vi "Main.vi"() -> ()   [LabVIEW 2017]
doc: "The myRIO Project template acquires acceleration data from the onboard accelerometer and displays the changes of acceleration values in a waveform chart."
uses:
  <vilib>/myRIO/Instrument Drivers/Onboard IO/AI/typedefs/AI Reference.ctl
  <vilib>/myRIO/Common/Instrument Driver Framework/Utilities/typedefs/myRIO Generic Hardware Reference.ctl
  <vilib>/myRIO/Common/Instrument Driver Framework/Utilities/typedefs/Hardware Version Enum.ctl
  <vilib>/myRIO/Common/Instrument Driver Framework/Utilities/typedefs/myRIO v1.0 Reference.ctl
  <vilib>/myRIO/Common/Instrument Driver Framework/Utilities/typedefs/Generic FPGA Reference.ctl
  <vilib>/myRIO/Common/Instrument Driver Framework/myRIO v1.0/AI/typedefs/AI Channels List.ctl
  <vilib>/myRIO/Common/Instrument Driver Framework/myRIO v1.0/AI/typedefs/AI Channels Enum.ctl
  <vilib>/myRIO/Common/Instrument Driver Framework/Utilities/typedefs/Analog Scaling Constants List.ctl
  <vilib>/myRIO/Common/Instrument Driver Framework/Utilities/typedefs/Analog Scaling Constants.ctl
  <vilib>/userdefined/High Color/nirio_resource_hc.ctl
  <vilib>/myRIO/Instrument Drivers/Onboard IO/DIO/typedefs/DIO Reference.ctl
  <vilib>/myRIO/Common/Instrument Driver Framework/myRIO v1.0/DIO/typedefs/DIO Channels List.ctl
  <vilib>/myRIO/Common/Instrument Driver Framework/myRIO v1.0/DIO/typedefs/DIO Channels Enum.ctl
  <vilib>/myRIO/Common/Instrument Driver Framework/Utilities/vis/Is FPGA Ref Available.vi
  <vilib>/myRIO/Common/Instrument Driver Framework/myRIO v1.0/AI/vis/myRIO v1.1 Open AI.vi
  <vilib>/myRIO/Instrument Drivers/Onboard IO/AI/vis/Read.vi
  <vilib>/Analysis/baseanly.llb/Mean (DBL).vi
  <vilib>/myRIO/Common/Instrument Driver Framework/myRIO v1.0/DIO/vis/myRIO v1.1 Open DIO.vi
  <vilib>/myRIO/Instrument Drivers/Onboard IO/DIO/vis/Write.vi
  <vilib>/myRIO/Common/Instrument Driver Framework/Utilities/vis/Validate Channels.vi
  <vilib>/myRIO/Common/Instrument Driver Framework/myRIO v1.0/AI/vis/myRIO v1.0 Reserve AI.vi
  <vilib>/myRIO/Common/Instrument Driver Framework/myRIO v1.0/DIO/vis/myRIO v1.0 Reserve DIO.vi
  <vilib>/myRIO/Common/Instrument Driver Framework/myRIO v1.0/UART/vis/myRIO v1.0 Close UART.vi
  <vilib>/myRIO/Common/Instrument Driver Framework/myRIO v1.0/AI/vis/myRIO v1.0 Build MUX Configuration AI.vi
  <vilib>/myRIO/Common/Instrument Driver Framework/myRIO v1.0/Resource Manager/vis/myRIO v1.0 Reserve Channel List.vi
  <vilib>/myRIO/Common/Instrument Driver Framework/myRIO v1.0/DIO/vis/myRIO v1.0 Build MUX Configuration DIO.vi
  <vilib>/myRIO/Common/Instrument Driver Framework/myRIO v1.0/Resource Manager/vis/myRIO v1.0 Reserve Channel.vi
  <vilib>/myRIO/Common/Instrument Driver Framework/myRIO v1.0/Resource Manager/vis/myRIO v1.0 Unreserve Channel.vi
  <vilib>/myRIO/Common/Instrument Driver Framework/myRIO v1.0/Resource Manager/vis/myRIO v1.0 Create Configuration List.vi
  <vilib>/myRIO/Common/Instrument Driver Framework/myRIO v1.0/Resource Manager/vis/myRIO v1.0 Build Mutex Name.vi
  <vilib>/Utility/VariantDataType/GetNumericInfo.vi
  <vilib>/Utility/error.llb/Error Cluster From Error Code.vi
  <vilib>/myRIO/Common/Instrument Driver Framework/myRIO v1.0/myRIO v1.1 Open.vi
  <vilib>/myRIO/Common/Instrument Driver Framework/myRIO v1.0/AI/vis/myRIO v1.0 Get Scaling Constants AI.vi
  <vilib>/myRIO/Common/Instrument Driver Framework/Utilities/vis/IO Manager.vi
  <vilib>/myRIO/Common/Instrument Driver Framework/Utilities/vis/Configuration Manager.vi
  <vilib>/myRIO/Common/Instrument Driver Framework/myRIO v1.0/myRIO v1.0 Close.vi
  <vilib>/myRIO/Common/Instrument Driver Framework/myRIO v1.0/AI/vis/myRIO v1.0 Read AI.vi
  <vilib>/myRIO/Common/Instrument Driver Framework/myRIO v1.0/Resource Manager/vis/myRIO v1.0 Configure IO.vi
  <vilib>/myRIO/Common/Instrument Driver Framework/myRIO v1.0/DIO/vis/myRIO v1.0 Write DIO.vi
  <vilib>/myRIO/Common/Instrument Driver Framework/Utilities/vis/FPGA Ref Manager.vi
  <vilib>/myRIO/Common/Instrument Driver Framework/myRIO v1.0/myRIO v1.0 Reset FPGA.vi
  <vilib>/myRIO/Common/Instrument Driver Framework/myRIO v1.0/IRQ/vis/myRIO v1.0 IRQ Info FGV.vi
  <vilib>/myRIO/Common/Instrument Driver Framework/myRIO v1.0/IRQ/vis/myRIO v1.0 Timer IRQ Info FGV.vi
  <vilib>/myRIO/Common/Instrument Driver Framework/myRIO v1.0/IRQ/vis/myRIO v1.0 ISR Agent.vi
  <vilib>/myRIO/Express VI/Onboard IO/AI/AI Express VI.xnode
  <vilib>/myRIO/Instrument Drivers/Onboard IO/AI/vis/myRIO AI Open.xnode
  <vilib>/myRIO/Express VI/Onboard Devices/LED/LED Express VI.xnode
  <vilib>/myRIO/Instrument Drivers/Onboard IO/DIO/vis/myRIO DIO Open.xnode
  <vilib>/myRIO/Instrument Drivers/Utilities/Utilities.lvlib
  <vilib>/myRIO/Instrument Drivers/Onboard IO/AI/AI.lvlib
  <vilib>/Analysis/NI_AALBase.lvlib
  <vilib>/myRIO/Instrument Drivers/Onboard IO/DIO/DIO.lvlib
panel:
  in  "LED Threthhold":dbl=0.45 format="%#_13g"
  in  "Points to Smooth":dbl=100.0 format="%#_13g"
  out "Moving Avg / Smoothed Waveform":waveform(dbl)(graph)
  out "Rectified Waveform Graph":waveform(dbl)(graph)
  out "Mean of Initialization Phase":dbl
  out "Waveform Graph":waveform(dbl)(graph)
  out "error out":errorcluster
  in  "Stop":bool
  # "ELEC3800: IoT                                               Lab06                                          Matt Bennett\nFall 2017                                                                                                               09/18/17"
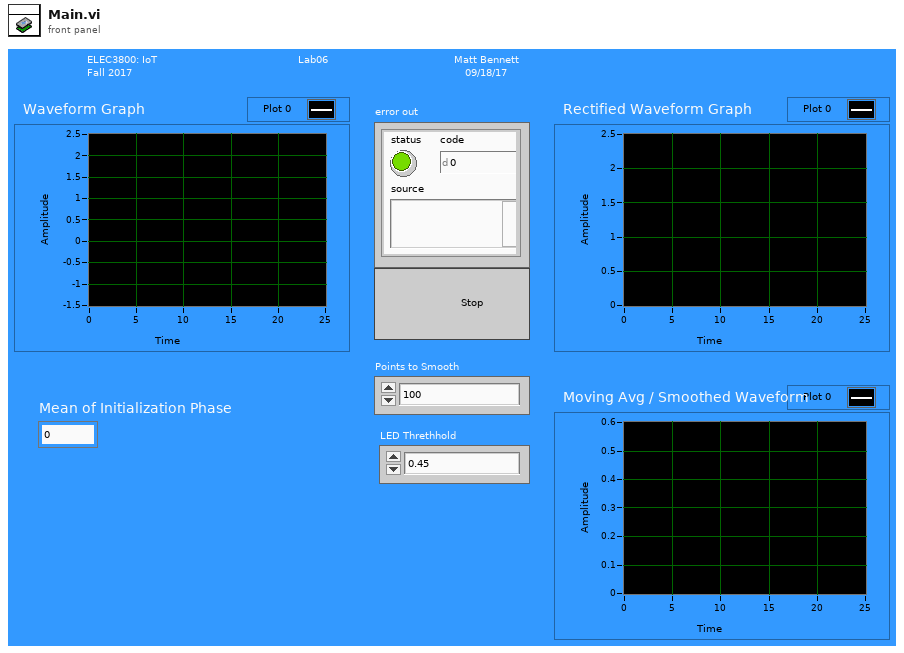
[diagram p1: front panel]
types:
  T1 = typedef "DIO.lvlib/DIO Reference.ctl" = cluster{"myRIO Reference":T2, "DIO Channels List":T6}
  T2 = typedef "myRIO Generic Hardware Reference.ctl" = cluster{"myRIO Model":T3, "myRIO Hardware Reference":T4}
  T3 = typedef "Hardware Version Enum.ctl" = enum16{"Unknown", "myRIO-1900", "myRIO-1950", "roboRIO", "NI ELVIS RIO CM"}
  T4 = typedef "myRIO v1.0 Reference.ctl" = cluster{"Generic FPGA Reference":T5, "Allow multiple opens":bool}
  T5 = typedef "Generic FPGA Reference.ctl" = refnum<k20>
  T6 = typedef "DIO Channels List.ctl" = T7[]
  T7 = typedef "DIO Channels Enum.ctl" = enum16{"Not Connected", "C/DIO0", "C/DIO1", "C/DIO2", "C/DIO3", "C/DIO4", "C/DIO5", "C/DIO6", "C/DIO7", "A/DIO0", "A/DIO1", "A/DIO2", "A/DIO3", "A/DIO4", "A/DIO5", "A/DIO6", "A/DIO7", "A/DIO8", "A/DIO9", "A/DIO10", "A/DIO11", "A/DIO12", "A/DIO13", "A/DIO14", "A/DIO15", "B/DIO0", "B/DIO1", "B/DIO2", "B/DIO3", "B/DIO4", "B/DIO5", "B/DIO6", "B/DIO7", "B/DIO8", "B/DIO9", "B/DIO10", "B/DIO11", "B/DIO12", "B/DIO13", "B/DIO14", "B/DIO15", "LED0", "LED1", "LED2", "LED3", "Button0", "DIO/DIO0", "DIO/DIO1", "DIO/DIO2", "DIO/DIO3", "DIO/DIO4", "DIO/DIO5", "DIO/DIO6", "DIO/DIO7", "DIO/DIO8", "DIO/DIO9", "SPI/CS0", "SPI/CS1", "SPI/CS2", "SPI/CS3", "LED RADIO (Green)", "LED RADIO (Red)", "LED COMM (Green)", "LED COMM (Red)", "LED MODE (Green)", "LED MODE (Red)"}
  T8 = typedef "nirio_resource_hc.ctl" = tag
  T9 = typedef "AI.lvlib/AI Reference.ctl" = cluster{"myRIO Reference":T2, "AI Channels List":T10, "AI Scaling Constants List":T12}
  T10 = typedef "AI Channels List.ctl" = T11[]
  T11 = typedef "AI Channels Enum.ctl" = enum16{"Not Connected", "AudioIn/Left", "AudioIn/Right", "C/AI0", "C/AI1", "A/AI0", "A/AI1", "A/AI2", "A/AI3", "B/AI0", "B/AI1", "B/AI2", "B/AI3", "AI/AI0", "AI/AI1", "AI/AI2", "AI/AI3"}
  T12 = typedef "Analog Scaling Constants List.ctl" = T13[]
  T13 = typedef "Analog Scaling Constants.ctl" = cluster{"LSB Weight (Volts)":dbl, "Offset (Volts)":dbl, "Signed?":bool}
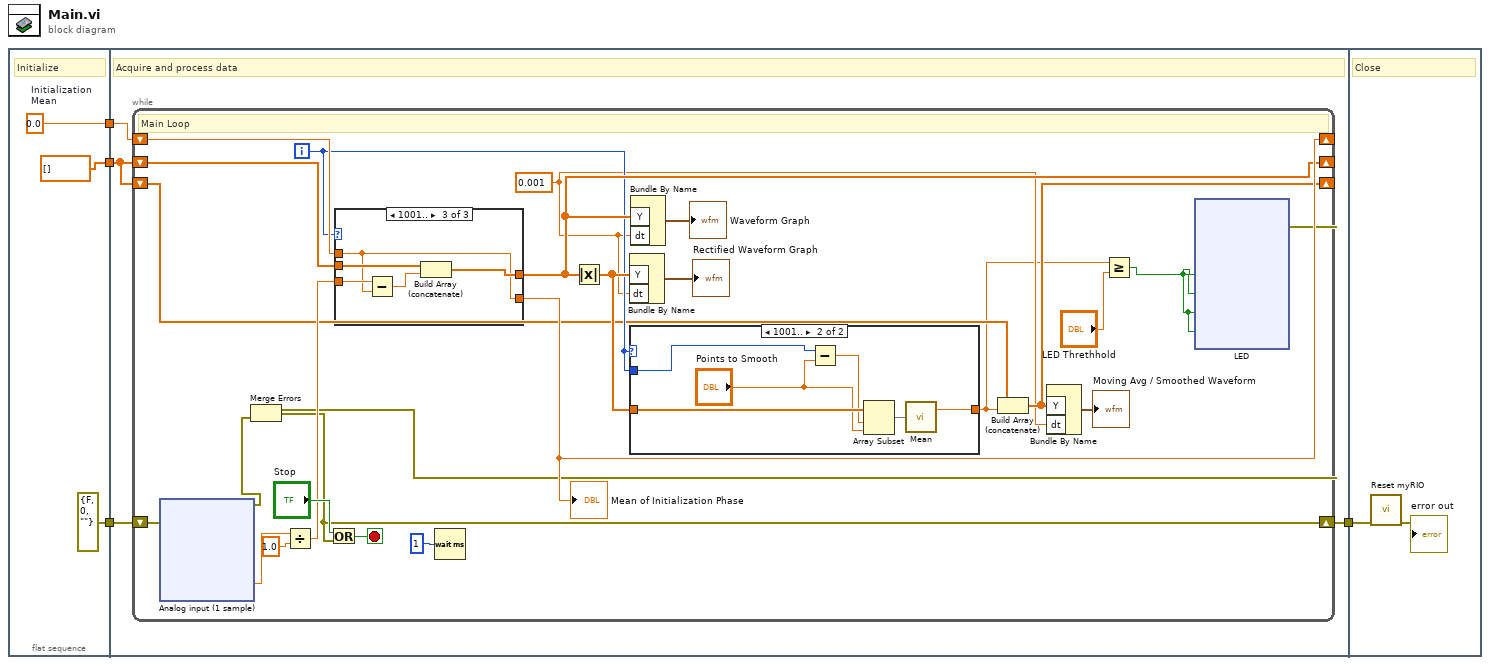
[diagram p0: block diagram]
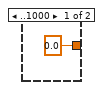
[diagram p2: hidden frame]
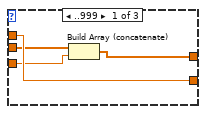
[diagram p3: hidden frame]
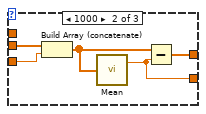
[diagram p4: hidden frame]
diagram:
  n1 = flat-sequence {
    tunnel: [errorcluster {"status"=FALSE, "code"=0, "source"=""} ("error in (no error)")] -> w4
    tunnel: [dbl[] []] -> w2
    tunnel: [w5] -> w1
    tunnel: w4 -> [w11]
    tunnel: [w10] -> w3
    tunnel: w2 -> [w8]
    tunnel: w1 -> [w9]
    tunnel: w3 -> [w134]
    frame #0 {
      w5 = 0.0  # Initialization  Mean
      # "Initialize"
    }
    frame #1 {
      # "Acquire and process data"
      n2 = while {
        shift-right: [w13] -> w10
        shift-left: w11 -> [w34]
        shift-right: [w24] -> _
        shift-left: w8 -> [w26]
        shift-right: [w27] -> _
        shift-left: w9 -> [w29]
        shift-right: [w19] -> _
        shift-left: w8 -> [w21]
        i -> [w22]
        stop <- w36 stop-if-true
        w18 = 0.001
        # "Main Loop"
        n3 = xnode "Analog input (1 sample)"("error in (no error)"=w34) -> ("C/AI0 (AI0)"=w32:dbl, "error out"=w14:errorcluster)
        n4 = Divide(x=w32, y=1.0) -> (x/y=w28:dbl)
        n5 = case shown="1001.." w22 {
          tunnel: [w82 w90 w93] -> w24
          tunnel: [w85 w89 w92] -> w27
          tunnel: w29 -> [w85 _ w92]
          tunnel: w26 -> [w84 w87 w94]
          tunnel: w28 -> [w83 w88 w95]
          frame ..999 {
            n6 = Build Array (concatenate)(w84, w83) -> (w82:dbl[])
          }
          frame 1000 {
            n7 = Build Array (concatenate)(w87, w88) -> (w86:dbl[])
            n8 = call-poly <vilib>:"Mean.vi"("X"=w86) -> ("mean"=w89:dbl)  [unwired: 1 out]
            n9 = Subtract(x=w86, y=w89) -> (x-y=w90:dbl[])
          }
          frame 1001.. {
            n10 = Subtract(x=w95, y=w92) -> (x-y=w91:dbl)
            n11 = Build Array (concatenate)(w94, w91) -> (w93:dbl[])
          }
        }
        "Mean of Initialization Phase" <- w27
        n12 = Wait (ms)(milliseconds to wait=1) -> ()  [unwired: 1 out]
        n13 = Absolute Value(x=w24) -> (abs(x)=w23:dbl[])
        n14 = Bundle By Name("Y"=w23, "dt"=w18) -> (→"Rectified Waveform Graph":waveform(dbl))  [unwired: 1 in]
        n15 = case shown="1001.." w22 {
          tunnel: w23 -> [_ w81]
          tunnel: [0.0 w76] -> w17
          tunnel: w22 -> [_ w79]
          frame ..1000 {
          }
          frame 1001.. {
            n16 = Subtract(x=w79, y="Points to Smooth") -> (x-y=w80:dbl)
            n17 = Array Subset(array=w81, index=w80, length="Points to Smooth") -> (w77:dbl[])
            n18 = call-poly <vilib>:"Mean.vi"("X"=w77) -> ("mean"=w76:dbl)  [unwired: 1 out]
          }
        }
        n19 = Bundle By Name("Y"=w24, "dt"=w18) -> (→"Waveform Graph":waveform(dbl))  [unwired: 1 in]
        n20 = Build Array (concatenate)(w21, w17) -> (w19:dbl[])
        n21 = Bundle By Name("Y"=w19, "dt"=w18) -> (→"Moving Avg / Smoothed Waveform":waveform(dbl))  [unwired: 1 in]
        n22 = Greater Or Equal?(x=w17, y="LED Threthhold") -> (x >= y?=w12:bool)
        n23 = xnode "LED"("LED0"=w12, "LED1"=w12, "LED2"=w12, "LED3"=w12) -> ("error out"=w15:errorcluster)  [unwired: 1 in]
        n24 = Merge Errors(w15, w14) -> (w13:errorcluster)
        n25 = Or(x="Stop", y=w13) -> (x .or. y?=w36:bool)
      }
    }
    frame #2 {
      # "Close"
      n26 = call <vilib>:"Reset myRIO.vi"("error in (no error)"=w134) -> ("error out"=→"error out":errorcluster)  [unwired: 10 in]
    }
  }
